vi "contrast rotate V0.5.vi"(8 "error in (no error)":errorcluster, 9 "Position in":T1, 11 "Target Angle":cluster{"Angle":dbl, "speed":dbl}) -> (0 "error out":errorcluster, 1 "output cluster":T1)   [LabVIEW 2019]
uses:
  position cluster.ctl
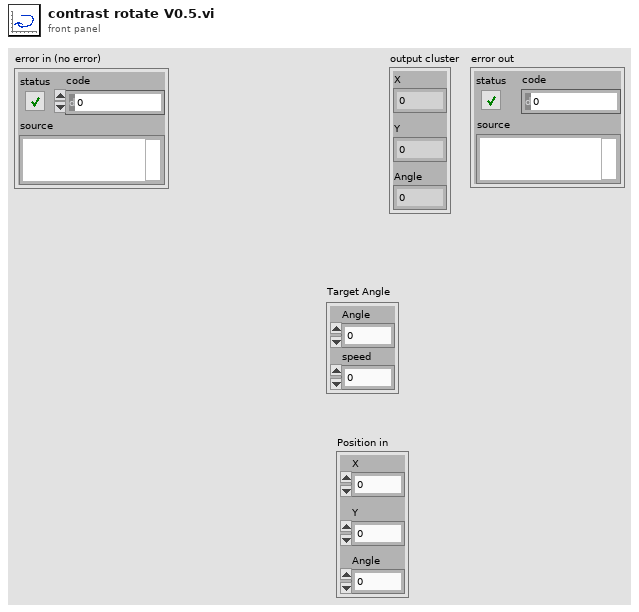
[diagram p1: front panel]
types:
  T1 = typedef "position cluster.ctl" = cluster{"X":dbl, "Y":dbl, "Angle":dbl}
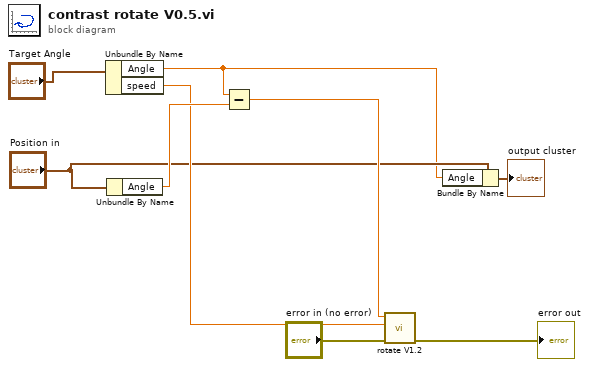
[diagram p0: block diagram]
diagram:
  n1 = Unbundle By Name("Target Angle") -> ("Angle"=w4:dbl, "speed"=w6:dbl)
  n2 = Unbundle By Name("Position in") -> ("Angle"=w8:dbl)
  n3 = Subtract(x=w4, y=w8) -> (x-y=w7:dbl)
  n4 = call "rotate V1.2.vi"("error in (no error)"="error in (no error)", "speed"=w6, "degree"=w7) -> ("error out"=→"error out":errorcluster)  [unwired: 8 in]
  n5 = Bundle By Name(cluster="Position in", "Angle"=w4) -> (→"output cluster":T1)
